vi "tttt_.vi"() -> ()   [LabVIEW 2020]
panel:
  out "Class Hierarchy 3":string[](array[string]) caption="类层次结构"
  out "Class Hierarchy 2":string[](array[string]) caption="类层次结构"
  out "Class Hierarchy":string[](array[string]) caption="类层次结构"
  out "数组 4":string[](array[string])
  out "大小":i32
  out "程序框图.所有对象[]":refnum<vi>[](array[refnum])
  out "数组 3":string[][](array[string])
  out "数组 2":string[](array[string])
  out "数组":string[](array[string])
  in  "Path to Entrance VI":path=path "C:/Users/Fred/Desktop/LabAI/main.vi"
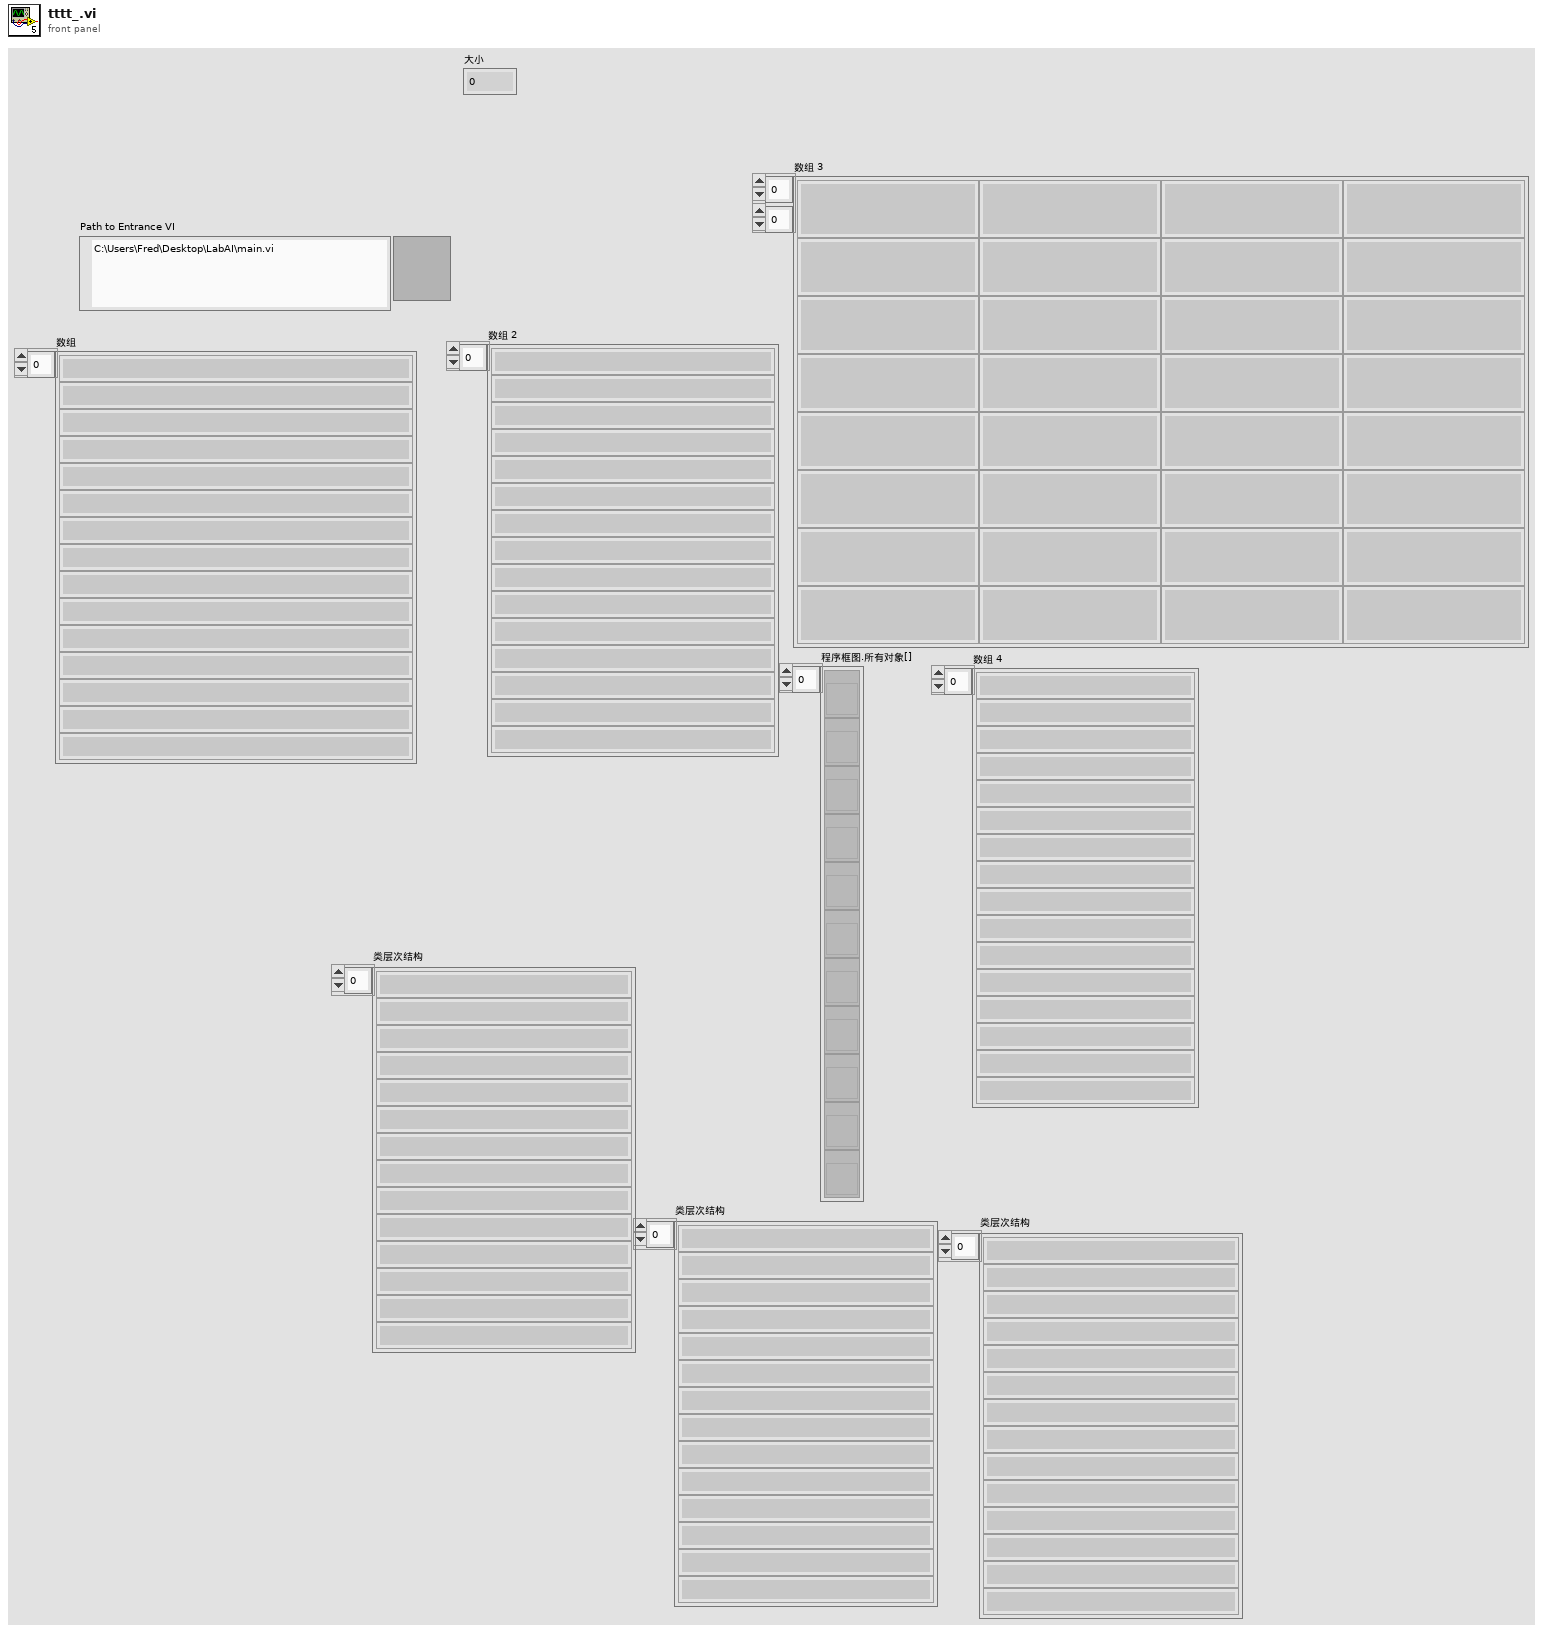
[diagram p1: front panel]
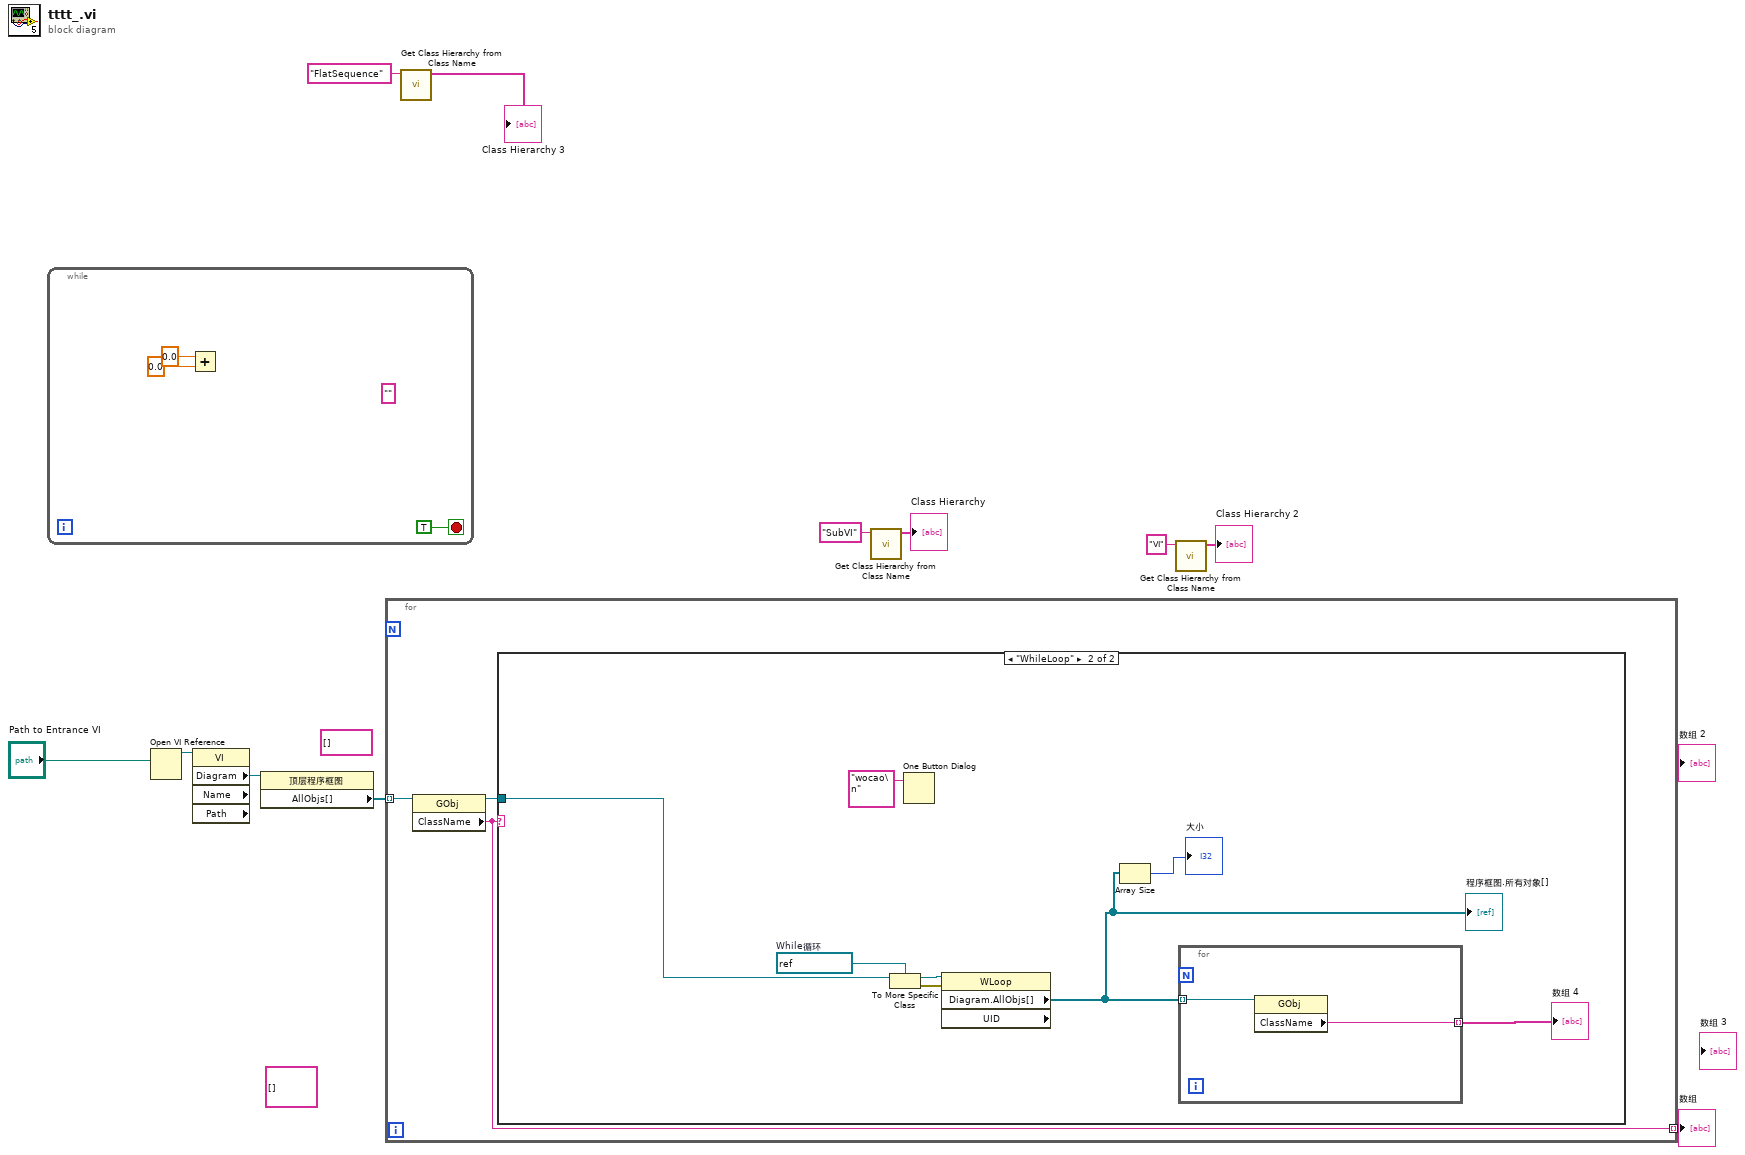
[diagram p0: block diagram]
diagram:
  (unwired) string[][] []
  (unwired) string[] []
  n1 = while {
    stop <- TRUE stop-if-true
    (unwired) ""
    n2 = Add(x=0.0, y=0.0) -> ()  [unwired: 1 out]
  }
  n3 = Open VI Reference(vi path="Path to Entrance VI") -> (vi reference=w10:refnum<vi>)  [unwired: 5 in, 1 out]
  n4 = property class="VI" props=["Diagram", "Name", "Path"](reference=w10) -> ("Diagram"=w8:refnum<vi>)  [unwired: 1 in, 4 out]
  n5 = property class="顶层程序框图"(reference=w8) -> ("AllObjs[]"=w7:refnum<vi>[])  [unwired: 1 in, 2 out]
  n6 = for {
    tunnel: [w16] -> w9 mode=indexing
    tunnel: w7 -> [w17] mode=indexing
    n7 = property class="GObj"(reference=w17) -> (reference out=w15:refnum<vi>, "ClassName"=w16:string)  [unwired: 1 in, 1 out]
    n8 = case shown="\"WhileLoop\"" w16 {
      tunnel: w15 -> [_ w22]
      frame "假", Default {
      }
      frame "WhileLoop" {
        w23 = refnum<vi> refnum  # While循环
        n9 = To More Specific Class(target class=w23, reference=w22) -> (specific class reference=w25:refnum<vi>, error out=w24:errorcluster)  [unwired: 1 in]
        n10 = One Button Dialog(message="wocao\n" ("消息")) -> ()  [unwired: 1 in, 1 out]
        n11 = property class="WLoop" props=["Diagram", "AllObjs[]", "UID"](reference=w25, error in=w24) -> ("Diagram.AllObjs[]"=w19:refnum<vi>[])  [unwired: 3 out]
        "程序框图.所有对象[]" <- w19
        n12 = Array Size(array=w19) -> (size(s)=→"大小":i32)
        n13 = for {
          tunnel: w19 -> [w27] mode=indexing
          tunnel: [w26] -> w18 mode=indexing
          n14 = property class="GObj"(reference=w27) -> ("ClassName"=w26:string)  [unwired: 1 in, 2 out]
        }
        "数组 4" <- w18
      }
    }
  }
  "数组" <- w9
  n15 = call <vilib>:"Get Class Hierarchy from Class Name.vi"("Class Name"="FlatSequence") -> ("Class Hierarchy"=→"Class Hierarchy 3":string[])  [unwired: 9 in, 1 out]
  n16 = call <vilib>:"Get Class Hierarchy from Class Name.vi"("Class Name"="SubVI") -> ("Class Hierarchy"=→"Class Hierarchy":string[])  [unwired: 9 in, 1 out]
  n17 = call <vilib>:"Get Class Hierarchy from Class Name.vi"("Class Name"="VI") -> ("Class Hierarchy"=→"Class Hierarchy 2":string[])  [unwired: 9 in, 1 out]
